vi "MainPTUdemo.vi"() -> ()   [LabVIEW 2019]
doc: "Read Binary File opens and reads an existing file stored as a double precision array in binary form. This VI shows the simplest way to read this entire file, with the simplest error checking."
panel:
  out "Processing:":i32
  out "GlobalResolution":dbl
  out "Resolution":dbl
  out "NumberOfRecords":i64
  out "TTTRRecType":i64 format="%x"
  out "n_hdr_items":i32=80
  out "Version":string
  out "Magic":string
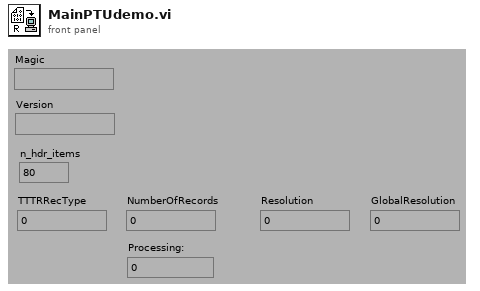
[diagram p1: front panel]
types:
  T1 = cluster{"TagIdent":string, "TagIndex":i32, "TagType":i32, "TagValue":i64, "TagAuxData":string}
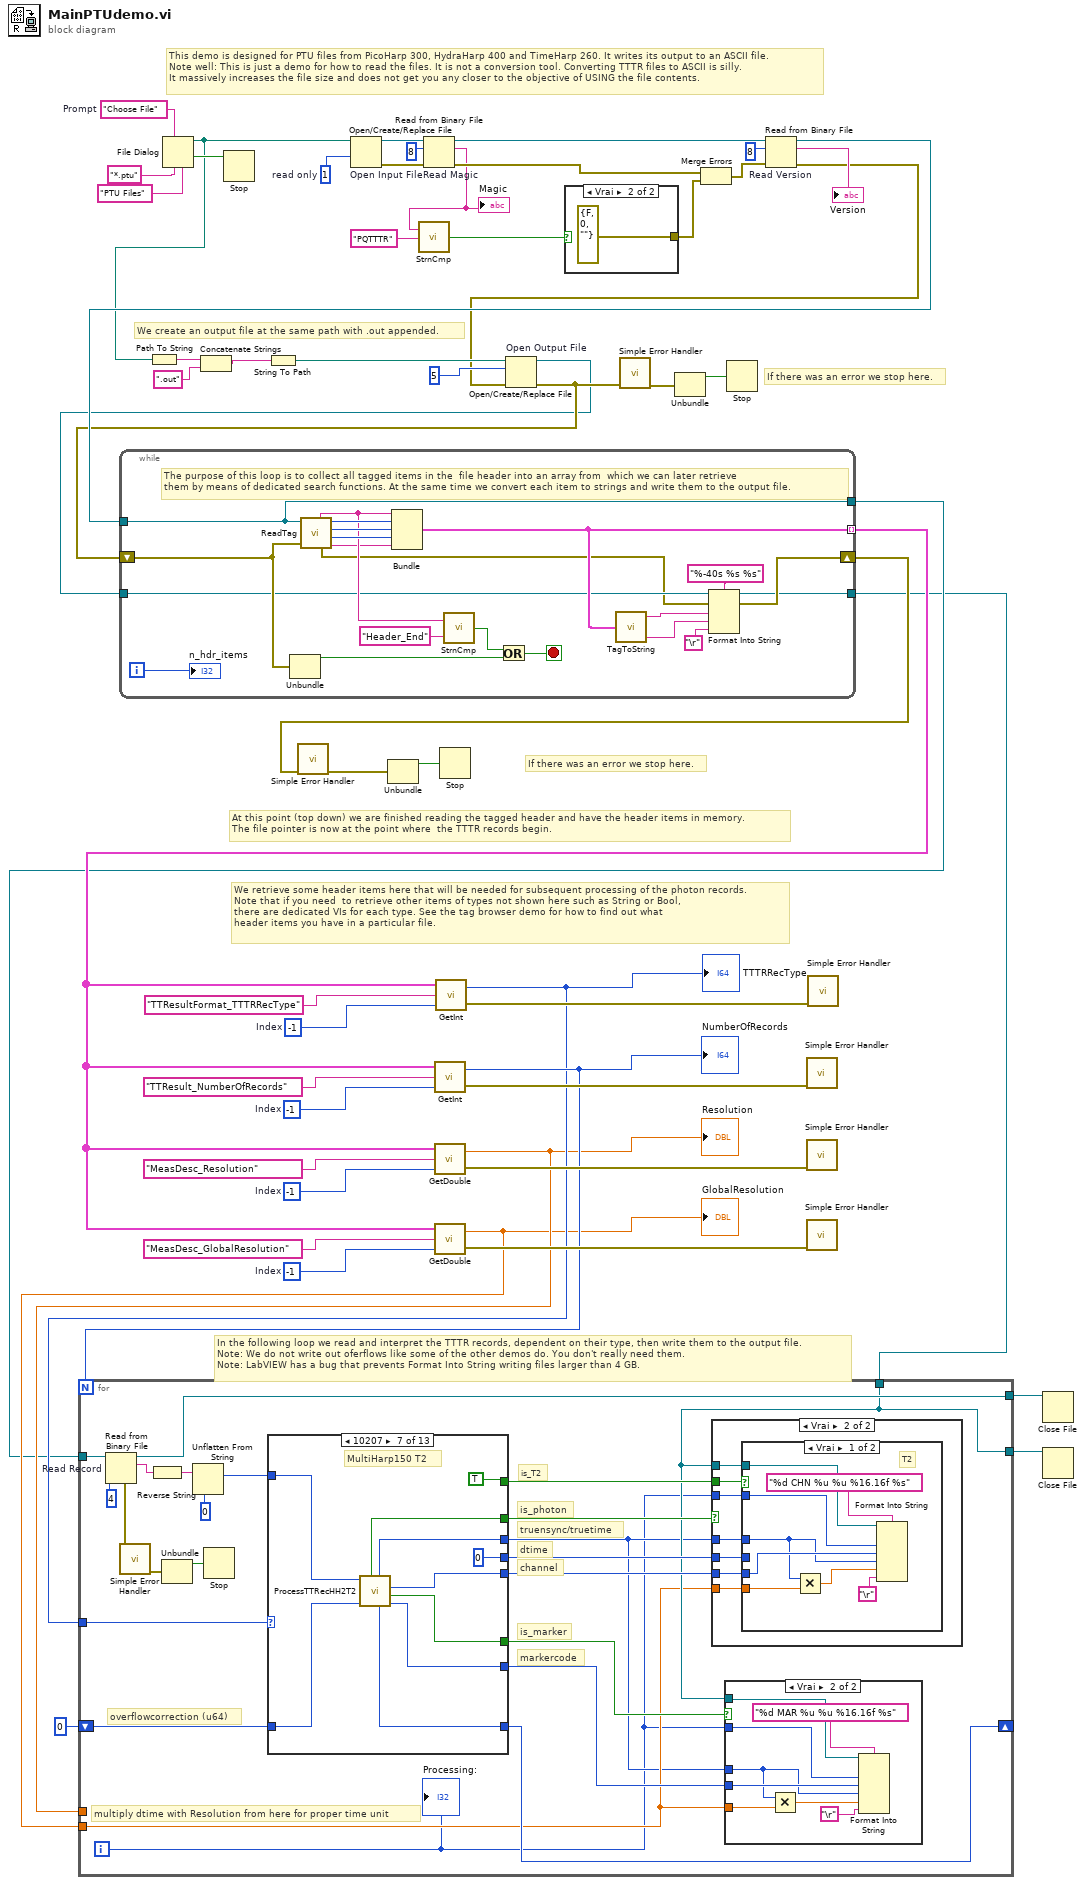
[diagram p0: block diagram]
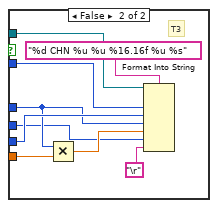
[diagram p4: hidden frame]
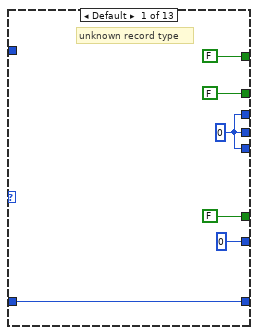
[diagram p5: hidden frame]
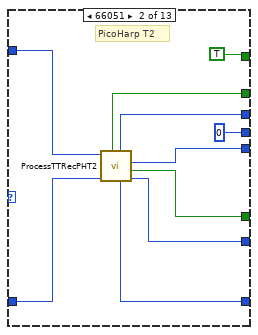
[diagram p6: hidden frame]
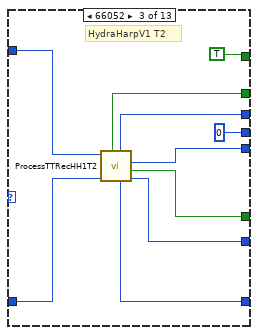
[diagram p7: hidden frame]
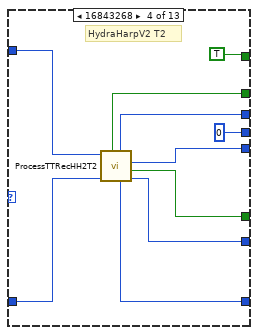
[diagram p8: hidden frame]
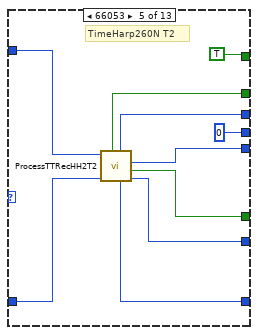
[diagram p9: hidden frame]
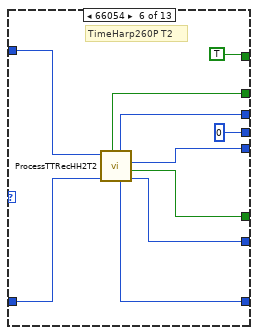
[diagram p10: hidden frame]
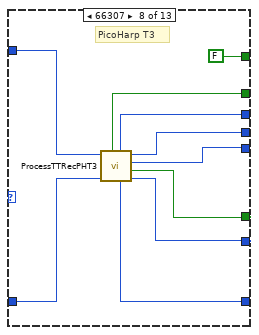
[diagram p11: hidden frame]
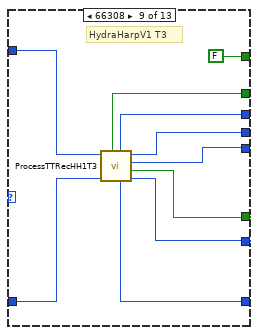
[diagram p12: hidden frame]
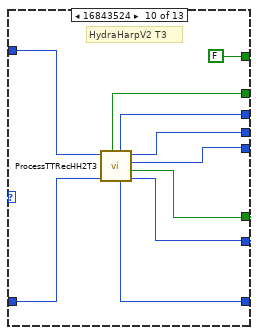
[diagram p13: hidden frame]
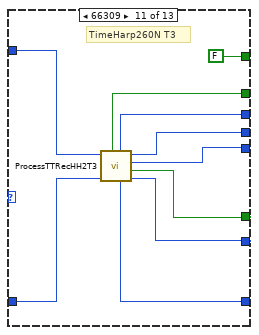
[diagram p14: hidden frame]
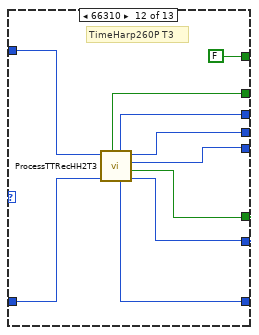
[diagram p15: hidden frame]
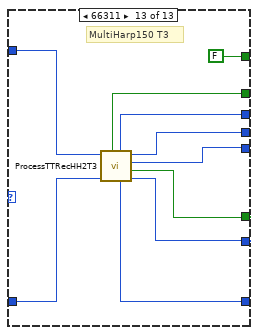
[diagram p16: hidden frame]
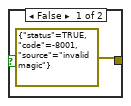
[diagram p17: hidden frame]
diagram:
  w13 = -1  # Index
  w30 = -1  # Index
  w33 = -1  # Index
  w36 = -1  # Index
  w1 = 1  # read only
  w54 = "Choose File"  # Prompt
  # "This demo is designed for PTU files from PicoHarp 300, HydraHarp 400 and TimeHarp 260. It writes its output to an ASCII file.\nNote well: This is just a demo for how to read the files. It is not a conversion tool. Converting TTTR files to ASCII is silly.\nIt massively increases the file size and does not get you any closer to the objective of USING the file contents."
  # "In the following loop we read and interpret the TTTR records, dependent on their type, then write them to the output file.\nNote: We do not write out oferflows like some of the other demos do. You don't really need them.\nNote: LabVIEW has a bug that prevents Format Into String writing files larger than 4 GB."
  # "If there was an error we stop here."
  # "We create an output file at the same path with .out appended."
  # "If there was an error we stop here."
  # "At this point (top down) we are finished reading the tagged header and have the header items in memory.\nThe file pointer is now at the point where  the TTTR records begin."
  # "We retrieve some header items here that will be needed for subsequent processing of the photon records.\nNote that if you need  to retrieve other items of types not shown here such as String or Bool, \nthere are dedicated VIs for each type. See the tag browser demo for how to find out what \nheader items you have in a particular file."
  n1 = File Dialog(4:"PTU Files", 6:"*.ptu", 7:w54) -> (1:w40:bool, 3:w25:path)  [unwired: 4 in, 2 out]
  n2 = Path To String(path=w25) -> (string=w24:string)
  n3 = Concatenate Strings(w24, ".out" ("string")) -> (w22:string)
  n4 = Stop(stop? (T)=w40) -> ()
  n5 = String To Path(string=w22) -> (path=w21:path)
  n6 = Open/Create/Replace File "Open Input File"(file path (use dialog)=w25, access (0:read/write)=w1) -> (refnum out=w42:refnum<file>, error out=w41:errorcluster)  [unwired: 4 in, 1 out]
  n7 = Read from Binary File "Read Magic"(8:w41, 10:8, 11:w42) -> (0:w49:errorcluster, 2:w45:string, 3:w53:refnum<file>)  [unwired: 3 in, 1 out]
  "Magic" <- w45
  n8 = call "StrnCmp.vi"("String 2"="PQTTTR", "String 1"=w45) -> ("equal"=w46:bool)
  n9 = case shown="Vrai" w46 {
    tunnel: [errorcluster {"status"=TRUE, "code"=-8001, "source"="invalid magic"} ("file error status 2") errorcluster {"status"=FALSE, "code"=0, "source"=""} ("file error status 2")] -> w47
    frame False {
    }
    frame True {
    }
  }
  n10 = Merge Errors(w49, w47) -> (w48:errorcluster)
  n11 = Read from Binary File "Read Version"(8:w48, 10:8, 11:w53) -> (0:w18:errorcluster, 2:→"Version":string, 3:w39:refnum<file>)  [unwired: 3 in, 1 out]
  n12 = Open/Create/Replace File "Open Output File"(file path (use dialog)=w21, error in=w18, operation (0:open)=5) -> (refnum out=w15:refnum<file>, error out=w17:errorcluster)  [unwired: 3 in, 1 out]
  n13 = while {
    shift-left: w17 -> [w76]
    shift-right: [w62] -> w28
    tunnel: w39 -> [w58]
    tunnel: [w66] -> w11 mode=indexing
    tunnel: w15 -> [w65]
    tunnel: [w59] -> w2
    tunnel: [w58] -> w6
    i -> [w72]
    stop <- w77 stop-if-true
    # "The purpose of this loop is to collect all tagged items in the  file header into an array from  which we can later retrieve \nthem by means of dedicated search functions. At the same time we convert each item to strings and write them to the output file."
    n14 = Unbundle(w76) -> ("status"=w69:bool)  [unwired: 2 out]
    n15 = call "ReadTag.vi"("refnum"=w58, "error in"=w76) -> ("TagIdent"=w68:string, "TagIndex"=w75:i32, "TagType"=w74:i32, "error out"=w63:errorcluster, "TagValue"=w73:i64, "TagAuxData"=w67:string)  [unwired: 3 in]
    n16 = Bundle("TagIdent"=w68, "TagIndex"=w75, "TagType"=w74, "TagValue"=w73, "TagAuxData"=w67) -> (w66:T1)  [unwired: 1 in]
    n17 = call "StrnCmp.vi"("String 2"="Header_End", "String 1"=w68) -> ("equal"=w70:bool)
    n18 = Or(x=w70, y=w69) -> (x .or. y?=w77:bool)
    n19 = call "TagToString.vi"("TagData"=w66) -> ("StrTagValue"=w60:string, "StrTagName"=w61:string)  [unwired: 2 in, 1 out]
    n20 = Format Into String(format string="%-40s %s %s", initial string=w65, error in=w63, w61, w60, "\r") -> (resulting string=w59:refnum<file>, error out=w62:errorcluster)
    "n_hdr_items" <- w72
  }
  n21 = call <vilib>:"Simple Error Handler.vi"("error in (no error)"=w28) -> ("error out"=w27:errorcluster)  [unwired: 4 in, 4 out]
  n22 = Unbundle(w27) -> ("status"=w26:bool)  [unwired: 2 out]
  n23 = call "GetInt.vi"("Index"=w33, "Ident"="TTResult_NumberOfRecords", "Array"=w11) -> ("error status"=w32:errorcluster, "TagValue"=w10:i64)
  "NumberOfRecords" <- w10
  n24 = call "GetDouble.vi"("Index"=w30, "Ident"="MeasDesc_Resolution", "Array"=w11) -> ("error status"=w29:errorcluster, "TagValue"=w8:dbl)
  "Resolution" <- w8
  n25 = call "GetDouble.vi"("Index"=w13, "Ident"="MeasDesc_GlobalResolution", "Array"=w11) -> ("error status"=w12:errorcluster, "TagValue"=w7:dbl)
  "GlobalResolution" <- w7
  n26 = call "GetInt.vi"("Index"=w36, "Ident"="TTResultFormat_TTTRRecType", "Array"=w11) -> ("error status"=w35:errorcluster, "TagValue"=w9:i64)
  "TTTRRecType" <- w9
  n27 = for {
    N: w10 -> [_]
    tunnel: w9 -> [w94]
    tunnel: w8 -> [_]
    tunnel: w7 -> [w81]
    tunnel: w6 -> [w96]
    tunnel: [w95] -> w5
    shift-right: [w83] -> _
    shift-left: u64 0 -> [w90]
    tunnel: [w84] -> w3
    tunnel: w2 -> [w84]
    i -> [w79]
    # "multiply dtime with Resolution from here for proper time unit"
    # "channel"
    # "dtime"
    # "truensync/truetime"
    # "is_T2"
    # "is_photon"
    # "markercode"
    # "is_marker"
    # "overflowcorrection (u64)"
    n28 = Read from Binary File "Read Record"(10:4, 11:w96) -> (0:w91:errorcluster, 2:w99:string, 3:w95:refnum<file>)  [unwired: 4 in, 1 out]
    n29 = call <vilib>:"Simple Error Handler.vi"("error in (no error)"=w91) -> ("error out"=w93:errorcluster)  [unwired: 4 in, 4 out]
    n30 = Reverse String(1:w99) -> (0:w100:string)
    n31 = Unbundle(w93) -> ("status"=w92:bool)  [unwired: 2 out]
    n32 = Unflatten From String(type=u32 0, binary string=w100) -> (value=w78:u32)  [unwired: 3 in, 2 out]
    n33 = Stop(stop? (T)=w92) -> ()
    n34 = case shown="10207" w94 {
      tunnel: w90 -> [w138 w147 w157 w167 w177 w187 w197 w207 w217 w227 w237 w247 w257]
      tunnel: [w138 w146 w156 w166 w176 w186 w196 w206 w216 w226 w236 w246 w256] -> w83
      tunnel: [FALSE w145 w155 w165 w175 w185 w195 w204 w214 w224 w234 w244 w254] -> w85
      tunnel: [u32 0 w144 w154 w164 w174 w184 w194 w205 w215 w225 w235 w245 w255] -> w82
      tunnel: [FALSE w141 w151 w161 w171 w181 w191 w201 w211 w221 w231 w241 w251] -> w89
      tunnel: [FALSE TRUE TRUE TRUE TRUE TRUE TRUE FALSE FALSE FALSE FALSE FALSE FALSE] -> w88
      tunnel: [w133 w142 w152 w162 w172 w182 w192 w202 w212 w222 w232 w242 w252] -> w80
      tunnel: [w133 0 0 0 u32 0 u32 0 u32 0 w199 w209 w219 w229 w239 w249] -> w87
      tunnel: [w133 w143 w153 w163 w173 w183 w193 w203 w213 w223 w233 w243 w253] -> w86
      tunnel: w78 -> [_ w148 w158 w168 w178 w188 w198 w200 w210 w220 w230 w240 w250]
      frame Default {
        w133 = u32 0
        # "unknown record type"
      }
      frame 66051 {
        # "PicoHarp T2"
        n35 = call "ProcessTTRecPHT2.vi"("oflcorr_in"=w147, "rawbits"=w148) -> ("markercode"=w144:u32, "is_marker"=w145:bool, "channel"=w143:u32, "oflcorr_out"=w146:u64, "truetime"=w142:u64, "is_photon"=w141:bool)  [unwired: 4 in]
      }
      frame 66052 {
        # "HydraHarpV1 T2"
        n36 = call "ProcessTTRecHH1T2.vi"("oflcorr_in"=w157, "rawbits"=w158) -> ("markercode"=w154:u32, "is_marker"=w155:bool, "channel"=w153:u32, "oflcorr_out"=w156:u64, "truetime"=w152:u64, "is_photon"=w151:bool)  [unwired: 4 in]
      }
      frame 16843268 {
        # "HydraHarpV2 T2"
        n37 = call "ProcessTTRecHH2T2.vi"("oflcorr_in"=w167, "rawbits"=w168) -> ("markercode"=w164:u32, "is_marker"=w165:bool, "channel"=w163:u32, "oflcorr_out"=w166:u64, "truetime"=w162:u64, "is_photon"=w161:bool)  [unwired: 4 in]
      }
      frame 66053 {
        # "TimeHarp260N T2"
        n38 = call "ProcessTTRecHH2T2.vi"("oflcorr_in"=w177, "rawbits"=w178) -> ("markercode"=w174:u32, "is_marker"=w175:bool, "channel"=w173:u32, "oflcorr_out"=w176:u64, "truetime"=w172:u64, "is_photon"=w171:bool)  [unwired: 4 in]
      }
      frame 66054 {
        # "TimeHarp260P T2"
        n39 = call "ProcessTTRecHH2T2.vi"("oflcorr_in"=w187, "rawbits"=w188) -> ("markercode"=w184:u32, "is_marker"=w185:bool, "channel"=w183:u32, "oflcorr_out"=w186:u64, "truetime"=w182:u64, "is_photon"=w181:bool)  [unwired: 4 in]
      }
      frame 66055 {
        # "MultiHarp150 T2"
        n40 = call "ProcessTTRecHH2T2.vi"("oflcorr_in"=w197, "rawbits"=w198) -> ("markercode"=w194:u32, "is_marker"=w195:bool, "channel"=w193:u32, "oflcorr_out"=w196:u64, "truetime"=w192:u64, "is_photon"=w191:bool)  [unwired: 4 in]
      }
      frame 66307 {
        # "PicoHarp T3"
        n41 = call "ProcessTTRecPHT3.vi"("oflcorr_in"=w207, "rawbits"=w200) -> ("markercode"=w205:u32, "is_marker"=w204:bool, "channel"=w203:u32, "dtime"=w199:u32, "oflcorr_out"=w206:u64, "numsync"=w202:u64, "is_photon"=w201:bool)  [unwired: 3 in]
      }
      frame 66308 {
        # "HydraHarpV1 T3"
        n42 = call "ProcessTTRecHH1T3.vi"("oflcorr_in"=w217, "rawbits"=w210) -> ("markercode"=w215:u32, "is_marker"=w214:bool, "channel"=w213:u32, "dtime"=w209:u32, "oflcorr_out"=w216:u64, "numsync"=w212:u64, "is_photon"=w211:bool)  [unwired: 3 in]
      }
      frame 16843524 {
        # "HydraHarpV2 T3"
        n43 = call "ProcessTTRecHH2T3.vi"("oflcorr_in"=w227, "rawbits"=w220) -> ("markercode"=w225:u32, "is_marker"=w224:bool, "channel"=w223:u32, "dtime"=w219:u32, "oflcorr_out"=w226:u64, "numsync"=w222:u64, "is_photon"=w221:bool)  [unwired: 3 in]
      }
      frame 66309 {
        # "TimeHarp260N T3"
        n44 = call "ProcessTTRecHH2T3.vi"("oflcorr_in"=w237, "rawbits"=w230) -> ("markercode"=w235:u32, "is_marker"=w234:bool, "channel"=w233:u32, "dtime"=w229:u32, "oflcorr_out"=w236:u64, "numsync"=w232:u64, "is_photon"=w231:bool)  [unwired: 3 in]
      }
      frame 66310 {
        # "TimeHarp260P T3"
        n45 = call "ProcessTTRecHH2T3.vi"("oflcorr_in"=w247, "rawbits"=w240) -> ("markercode"=w245:u32, "is_marker"=w244:bool, "channel"=w243:u32, "dtime"=w239:u32, "oflcorr_out"=w246:u64, "numsync"=w242:u64, "is_photon"=w241:bool)  [unwired: 3 in]
      }
      frame 66311 {
        # "MultiHarp150 T3"
        n46 = call "ProcessTTRecHH2T3.vi"("oflcorr_in"=w257, "rawbits"=w250) -> ("markercode"=w255:u32, "is_marker"=w254:bool, "channel"=w253:u32, "dtime"=w249:u32, "oflcorr_out"=w256:u64, "numsync"=w252:u64, "is_photon"=w251:bool)  [unwired: 3 in]
      }
    }
    n47 = case shown="Vrai" w89 {
      tunnel: w88 -> [_ w115]
      tunnel: w80 -> [_ w112]
      tunnel: w87 -> [_ w109]
      tunnel: w86 -> [_ w113]
      tunnel: w79 -> [_ w114]
      tunnel: w81 -> [_ w111]
      tunnel: w84 -> [_ w110]
      frame False {
      }
      frame True {
        n48 = case shown="Vrai" w115 {
          tunnel: w114 -> [w122 w131]
          tunnel: w113 -> [w121 w130]
          tunnel: w112 -> [w119 w128]
          tunnel: w110 -> [w120 w129]
          tunnel: w111 -> [w118 w127]
          tunnel: w109 -> [_ w125]
          frame True {
            # "T2"
            n49 = Multiply(x=w119, y=w118) -> (x*y=w117:dbl)
            n50 = Format Into String(format string="%d CHN %u %u %16.16f %s", initial string=w120, w122, w121, w119, w117, "\r") -> ()  [unwired: 1 in, 2 out]
          }
          frame False {
            # "T3"
            n51 = Multiply(x=w128, y=w127) -> (x*y=w126:dbl)
            n52 = Format Into String(format string="%d CHN %u %u %16.16f %u %s", initial string=w129, w131, w130, w128, w126, w125, "\r") -> ()  [unwired: 1 in, 2 out]
          }
        }
      }
    }
    n53 = case shown="Vrai" w85 {
      tunnel: w79 -> [_ w107]
      tunnel: w84 -> [_ w106]
      tunnel: w82 -> [_ w104]
      tunnel: w81 -> [_ w102]
      tunnel: w80 -> [_ w101]
      frame False {
      }
      frame True {
        n54 = Multiply(x=w101, y=w102) -> (x*y=w103:dbl)
        n55 = Format Into String(format string="%d MAR %u %u %16.16f %s", initial string=w106, w107, w104, w101, w103, "\r") -> ()  [unwired: 1 in, 2 out]
      }
    }
    "Processing:" <- w79
  }
  n56 = Stop(stop? (T)=w26) -> ()
  n57 = call <vilib>:"Simple Error Handler.vi"("error in (no error)"=w17) -> ("error out"=w16:errorcluster)  [unwired: 4 in, 4 out]
  n58 = Unbundle(w16) -> ("status"=w19:bool)  [unwired: 2 out]
  n59 = Stop(stop? (T)=w19) -> ()
  n60 = call <vilib>:"Simple Error Handler.vi"("error in (no error)"=w32) -> ()  [unwired: 4 in, 5 out]
  n61 = call <vilib>:"Simple Error Handler.vi"("error in (no error)"=w29) -> ()  [unwired: 4 in, 5 out]
  n62 = call <vilib>:"Simple Error Handler.vi"("error in (no error)"=w12) -> ()  [unwired: 4 in, 5 out]
  n63 = call <vilib>:"Simple Error Handler.vi"("error in (no error)"=w35) -> ()  [unwired: 4 in, 5 out]
  n64 = Close File(refnum=w5) -> ()  [unwired: 1 in, 2 out]
  n65 = Close File(refnum=w3) -> ()  [unwired: 1 in, 2 out]
